vi "FOV_Zoom_Frame to Hex.vi"(5 "timings_offsets":dbl[](array[numeric]), 7 "distortion_corr":dbl, 8 "Objective":i8=20, 9 "Z pixel Size":i8=4, 11 "AOL_Globals":T1={"Imaging Protocol"=enum."AOL Z-Stack", "Number of POI"=0, "Number of Miniscans"=0, "Number of Trials"=0, "Number of Cycles "=0, "# Averaged Frames"=0, "Laser power (%)"=0, "Pockels (V)"=0.0, "Acquisition Length (sec)"=0.0, "Fill time (us)"=0.0, "POI Dwell time (us)"=0.0, "Miniscan Dwell time per pixel (us)"=0.0, "PMT 1"=0.0, "PMT 2"=0.0, "Back Apperture (mA)"=0.0, "Frame Size"=0, "Center Frequency"=0.0, "Field of View (norm)"=0.0, "DwellTime (us)"=0.0, "Wavelength (nm)"=0.0, "Zoom"=0.0, "AOL Z"=0.0, "AOL Mode"=enum."Raster", "GridXY"=0.0, "GridZ"=0.0, "TriggerPeriod (sec)"=0.0, "Number of Pixels in Miniscan"=0, "Experiment folder path"=path "", "X centre"=0.0, "Y centre"=0.0, "Angle (degrees)"=0.0, "Plane Mode"=0, "Threshold"=[], "Regenerate Chirps"=FALSE, "Rectangle ROI length (pixels)"=0, "Rectangle ROI height (pixels)"=0, "AOD fill"=4900, "StartupDelay"=0, "Samples Wait after Trigger"=5080, "Slip Cycle"=600000, "Add Cycle"=TRUE, "Functional Mode"=enum."Point", "Z Start"=0.0, "Z Stop"=0.0, "# Planes"=0} {"Plane Mode" items=["XY Plane", "XZ Plane", "YZ Plane", "arbitraryplane"]; "Frame Size" items=["100X100"=100, "128X128"=128, "200X200"=200, "256X256"=256, "512X512"=512, "1024x1024"=1024, "2048x2048"=2048]; "Back Apperture (mA)" format="%#.6g"; "Pockels (V)" format="%#.6g"; "PMT 2" format="%#.6g"; "PMT 1" format="%#.6g"; "Angle (degrees)" format="%#.6g"; "POI Dwell time (us)" format="%#.6g"}) -> (3 "FOV-Zoom-FrameSize Hex":string)   [LabVIEW 2017]
uses:
  Typedefs/Controls/AOL_Globals.ctl
  Typedefs/Imaging Protocols enum.ctl
  Typedefs/Frame Size.ctl
  Typedefs/AOL modes.ctl
  Typedefs/Plane Mode.ctl
  Typedefs/Functional Mode.ctl
  <vilib>/Utility/miscctls.llb/LVStringsAndValuesArrayTypeDef_SGL.ctl
panel:
  out "length":i32
  out "Field of view (um)":dbl
  # "SUBROUTINE"
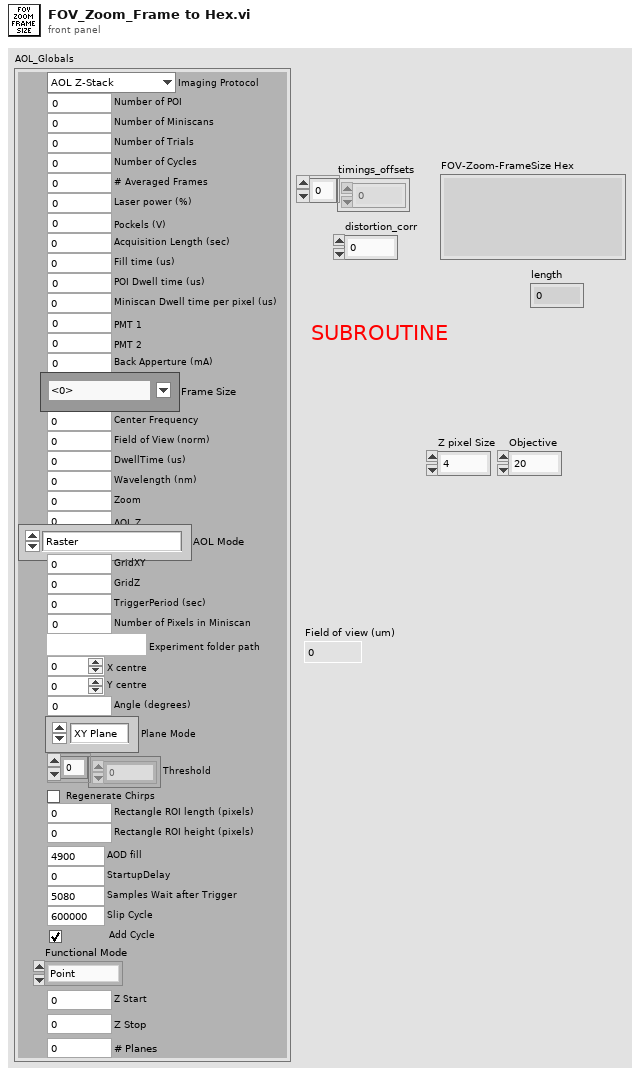
[diagram p1: front panel]
types:
  T1 = typedef "AOL_Globals.ctl" = cluster{"Imaging Protocol":T2, "Number of POI":u16, "Number of Miniscans":u16, "Number of Trials":u16, "Number of Cycles ":u64, "# Averaged Frames":u16, "Laser power (%)":u8, "Pockels (V)":dbl, "Acquisition Length (sec)":dbl, "Fill time (us)":dbl, "POI Dwell time (us)":dbl, "Miniscan Dwell time per pixel (us)":dbl, "PMT 1":dbl, "PMT 2":dbl, "Back Apperture (mA)":dbl, "Frame Size":T3, "Center Frequency":dbl, "Field of View (norm)":dbl, "DwellTime (us)":dbl, "Wavelength (nm)":dbl, "Zoom":dbl, "AOL Z":dbl, "AOL Mode":T4, "GridXY":dbl, "GridZ":dbl, "TriggerPeriod (sec)":dbl, "Number of Pixels in Miniscan":u16, "Experiment folder path":path, "X centre":dbl, "Y centre":dbl, "Angle (degrees)":dbl, "Plane Mode":T5, "Threshold":u16[], "Regenerate Chirps":bool, "Rectangle ROI length (pixels)":u16, "Rectangle ROI height (pixels)":u16, "AOD fill":u16, "StartupDelay":i32, "Samples Wait after Trigger":u16, "Slip Cycle":u32, "Add Cycle":bool, "Functional Mode":T6, "Z Start":dbl, "Z Stop":dbl, "# Planes":i32}
  T2 = typedef "Imaging Protocols enum.ctl" = enum16{"AOL Z-Stack", "Motor Z Stack", "Functional Acquisition", "Single Plane Acquisition", "Volume Acquisition", "Live Imaging", "Live Plane Imaging", "Live Volume Imaging"}
  T3 = typedef "Frame Size.ctl" = u16
  T4 = typedef "AOL modes.ctl" = enum16{"Raster", "Structural", "Pointing", "Mini Scan", "Alignment"}
  T5 = typedef "Plane Mode.ctl" = u16
  T6 = typedef "Functional Mode.ctl" = enum16{"Point", "Line", "Patch", "Plane", "Volume"}
  T7 = typedef "LVStringsAndValuesArrayTypeDef_SGL.ctl" = cluster{"String":string, "Value":sgl}[]
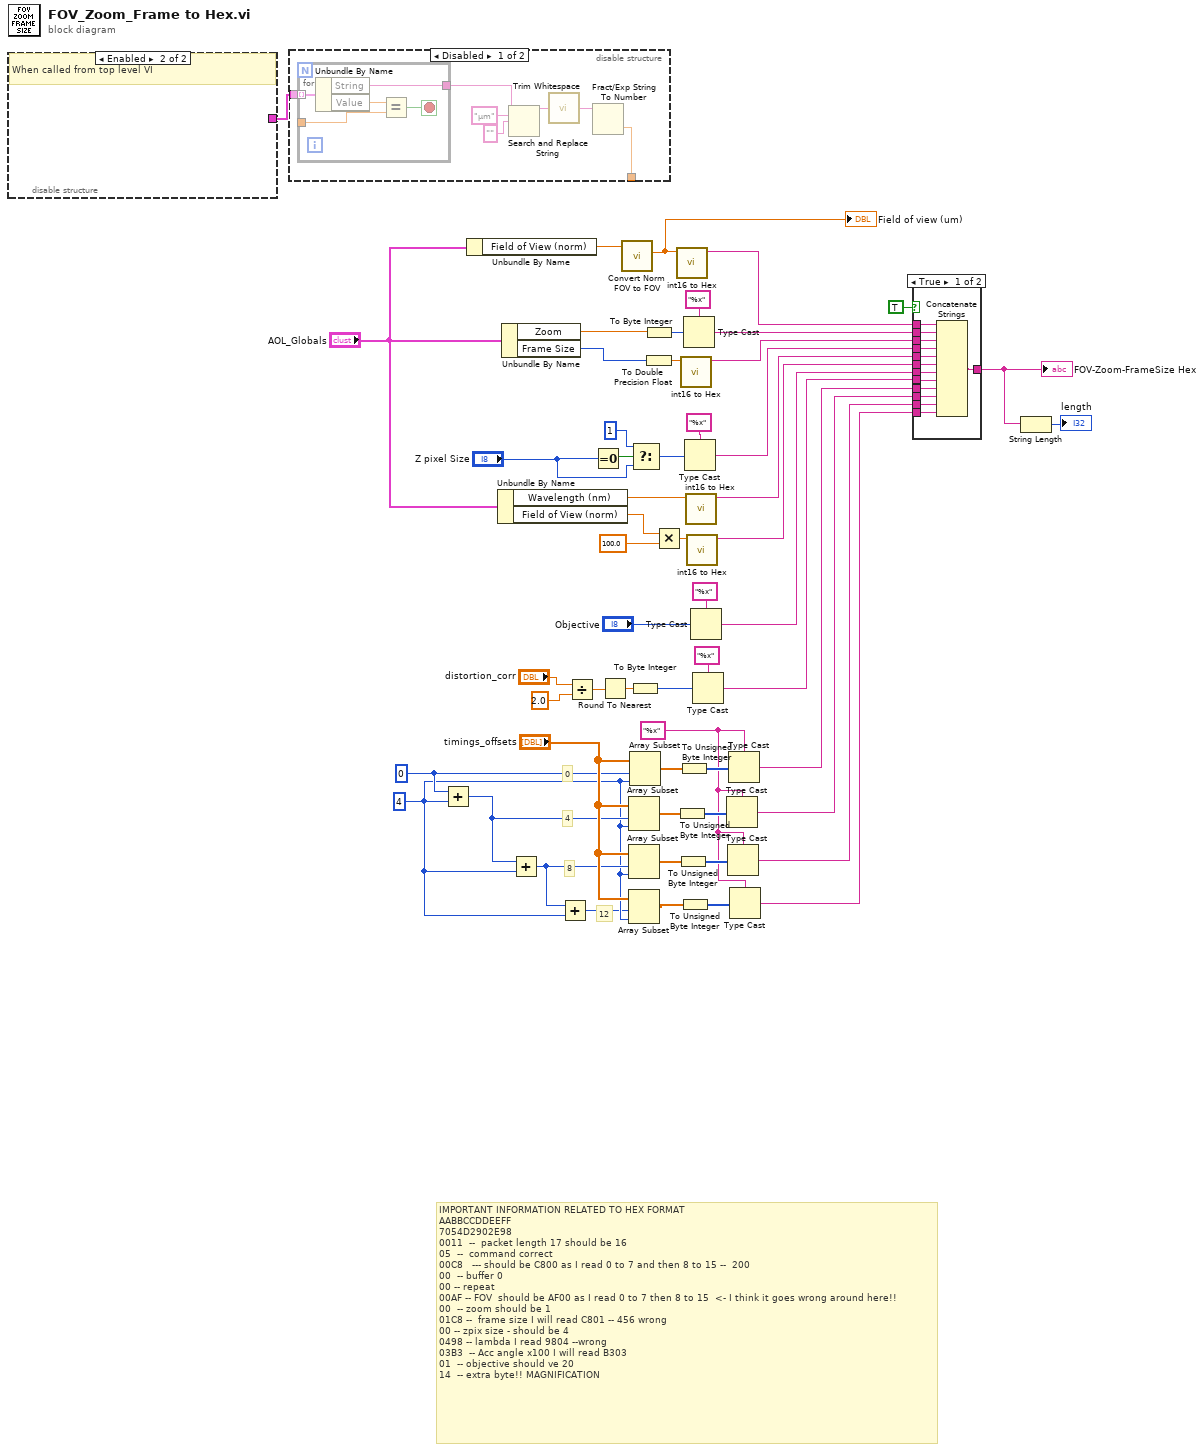
[diagram p0: block diagram]
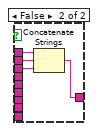
[diagram p3: hidden frame]
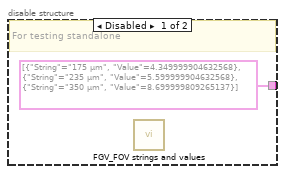
[diagram p4: hidden frame]
diagram:
  w7 = 4 ("y")
  w10 = 0 ("index")
  w15 = "%x" ("type")
  # "12"
  # "8"
  # "4"
  # "0"
  # "IMPORTANT INFORMATION RELATED TO HEX FORMAT\nAABBCCDDEEFF\n7054D2902E98\n0011  --  packet length 17 should be 16\n05  --  command correct\n00C8   --- should be C800 as I read 0 to 7 and then 8 to 15 --  200\n00  -- buffer 0\n00 -- repeat\n00AF -- FOV  should be AF00 as I read 0 to 7 then 8 to 15  <- I think it goes wrong around here!!\n00  -- zoom should be 1\n01C8 --  frame size I will read C801 -- 456 wrong\n00 -- zpix size - should be 4\n0498 -- lambda I read 9804 --wrong\n03B3  -- Acc angle x100 I will read B303\n01  -- objective should ve 20\n14  -- extra byte!! MAGNIFICATION"
  n1 = disable-structure shown="Enabled" {
    disable-tunnel: [T7 [{"String"="175 µm", "Value"=4.35}, {"String"="235 µm", "Value"=5.6}, {"String"="350 µm", "Value"=8.7}] ("Strings And Values []") _] -> w48
    frame Disabled {
      # "For testing standalone"
      n2 = call "FGV_FOV strings and values.vi"() -> ()  [unwired: 10 in, 2 out]
    }
    frame Enabled {
      # "When called from top level VI"
    }
  }
  n3 = disable-structure shown="Disabled" {
    disable-tunnel: [w59 _] -> _
    disable-tunnel: w48 -> [w58 _]
    frame Disabled {
      n4 = for {
        tunnel: _ -> [w67]
        tunnel: w58 -> [w69] mode=indexing
        tunnel: [w65] -> w60
        stop <- w66 stop-if-true
        n5 = Unbundle By Name(w69) -> ("String"=w65:string, "Value"=w68:sgl)
        n6 = Equal?(x=w68, y=w67) -> (x = y?=w66:bool)
      }
      n7 = Search and Replace String(input string=w60, search string="µm", replace string="" ("replace string (\"\")")) -> (result string=w63:string)  [unwired: 5 in, 3 out]
      n8 = call <vilib>:"Trim Whitespace.vi"("string"=w63) -> ("trimmed string"=w64:string)  [unwired: 1 in]
      n9 = Fract/Exp String To Number(string=w64) -> (number=w59:dbl)  [unwired: 3 in, 1 out]
    }
    frame Enabled {
    }
  }
  n10 = Add(x=w10, y=w7) -> (x+y=w9:i32)
  n11 = Unbundle By Name("AOL_Globals") -> ("Field of View (norm)"=w33:dbl)
  n12 = Unbundle By Name("AOL_Globals") -> ("Wavelength (nm)"=w47:dbl, "Field of View (norm)"=w45:dbl)
  n13 = Unbundle By Name("AOL_Globals") -> ("Zoom"=w52:dbl, "Frame Size"=w56:T3)
  n14 = Add(x=w9, y=w7) -> (x+y=w8:i32)
  n15 = Add(x=w8, y=w7) -> (x+y=w6:i32)
  n16 = Divide(x="distortion_corr", y=2.0) -> (x/y=w3:dbl)
  n17 = Equal To 0?(x="Z pixel Size") -> (x = 0?=w35:bool)
  n18 = Round To Nearest(number=w3) -> (nearest integer value=w2:dbl)
  n19 = call "Convert Norm FOV to FOV.vi"("Field of View(norm)"=w33) -> ("FOV"=w32:dbl)  [unwired: 10 in]
  "Field of view (um)" <- w32
  n20 = Array Subset(array="timings_offsets", index=w9, length=w7) -> (w20:dbl[])
  n21 = Array Subset(array="timings_offsets", index=w8, length=w7) -> (w16:dbl[])
  n22 = Array Subset(array="timings_offsets", index=w6, length=w7) -> (w17:dbl[])
  n23 = To Byte Integer(number=w2) -> (8bit integer=w25:i8)
  n24 = Array Subset(array="timings_offsets", index=w10, length=w7) -> (w23:dbl[])
  n25 = Select(t=i8 1, s=w35, f="Z pixel Size") -> (s? t:f=w36:i8)
  n26 = To Byte Integer(number=w52) -> (8bit integer=w53:i8)
  n27 = To Double Precision Float(number=w56) -> (double precision float=w55:dbl)
  n28 = Multiply(x=w45, y=100.0) -> (x*y=w46:dbl)
  n29 = call "int16 to Hex.vi"("number"=w32) -> ("Hex string"=w51:string)  [unwired: 10 in]
  n30 = To Unsigned Byte Integer(number=w20) -> (unsigned 8bit integer=w21:u8[])
  n31 = To Unsigned Byte Integer(number=w16) -> (unsigned 8bit integer=w19:u8[])
  n32 = To Unsigned Byte Integer(number=w23) -> (unsigned 8bit integer=w22:u8[])
  n33 = To Unsigned Byte Integer(number=w17) -> (unsigned 8bit integer=w18:u8[])
  n34 = call "int16 to Hex.vi"("number"=w55) -> ("Hex string"=w49:string)  [unwired: 10 in]
  n35 = Type Cast(type="%x", x=w53) -> (*(type *) &x=w50:string)
  n36 = Type Cast(type="%x", x=w36) -> (*(type *) &x=w41:string)
  n37 = call "int16 to Hex.vi"("number"=w47) -> ("Hex string"=w40:string)  [unwired: 10 in]
  n38 = call "int16 to Hex.vi"("number"=w46) -> ("Hex string"=w31:string)  [unwired: 10 in]
  n39 = Type Cast(type="%x", x="Objective") -> (*(type *) &x=w29:string)
  n40 = Type Cast(type="%x", x=w25) -> (*(type *) &x=w26:string)
  n41 = Type Cast(type=w15, x=w21) -> (*(type *) &x=w13:string)
  n42 = Type Cast(type=w15, x=w19) -> (*(type *) &x=w12:string)
  n43 = Type Cast(type=w15, x=w22) -> (*(type *) &x=w14:string)
  n44 = Type Cast(type=w15, x=w18) -> (*(type *) &x=w11:string)
  n45 = case shown="True" TRUE {
    tunnel: w51 -> [w82 w86]
    tunnel: w50 -> [w81 w85]
    tunnel: w49 -> [w80 w84]
    tunnel: [w79 w83] -> w27
    tunnel: w41 -> [w78 _]
    tunnel: w40 -> [w77 _]
    tunnel: w31 -> [w76 _]
    tunnel: w29 -> [w75 _]
    tunnel: w26 -> [w74 _]
    tunnel: w14 -> [w73 _]
    tunnel: w13 -> [w72 _]
    tunnel: w12 -> [w71 _]
    tunnel: w11 -> [w70 _]
    frame True {
      n46 = Concatenate Strings(w82, w81, w80, w78, w77, w76, w75, w74, w73, w72, w71, w70) -> (w79:string)
    }
    frame False {
      n47 = Concatenate Strings(w86, w85, w84) -> (w83:string)
    }
  }
  "FOV-Zoom-FrameSize Hex" <- w27
  n48 = String Length(string=w27) -> (length=→"length":i32)
